vi "Receive Value Change Event.vi"(8 "error in (no error)":errorcluster, 10 "ValueChangeMsg":refnum<class "ValueChangeMsg.lvclass">, 11 "Login View In":refnum<class "Login View.lvclass">) -> (0 "error out":errorcluster, 3 "Login View Out":refnum<class "Login View.lvclass">)   [LabVIEW 2017, in "Login View.lvlib" / "Login View.lvclass"]
doc: "<License>\nCopyright © 2017 Composed Systems, LLC | All rights reserved\nwww.composed.io\n\nAuthor: Ethan Stern <ethan.stern@composed.io>\n\nThis software is provided \"AS IS\" WITHOUT WARRANTIES, either express or implied, AND IS FOR EDUCATIONAL PURPOSES ONLY.\n</License>"
uses:
  Login View.lvclass
  <vilib>/gpm_packages/@cs/mva-viewable/Source/ActorEvents/IEventAggregator Messages/ValueChangeMsg/ValueChangeMsg.lvclass
  <vilib>/gpm_packages/@cs/mva-viewable/Source/ActorEvents/IEventAggregator Messages/ValueChangeMsg/ValueChangeMsg.lvclass/ValueChangeMsg.ctl
  Login View.lvclass/Login View.ctl
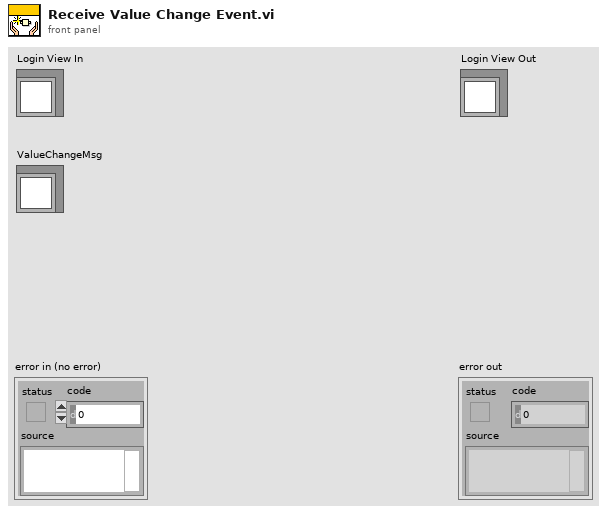
[diagram p1: front panel]
types:
  T1 = typedef "User Manager Application Types.lvlib/Credentials.ctl" = cluster{"Username":string, "Password":string}
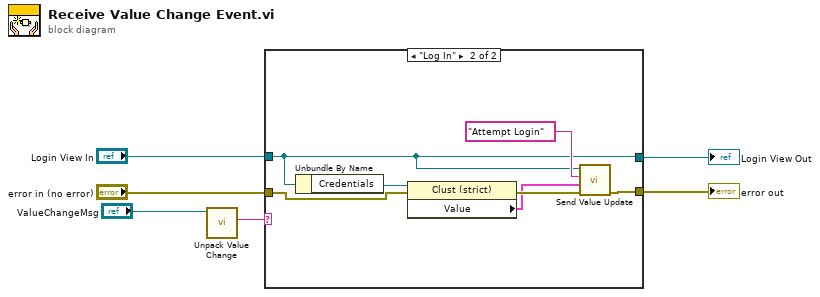
[diagram p0: block diagram]
diagram:
  n1 = call <vilib>:"Unpack Value Change.vi"("ValueChangeMsg"="ValueChangeMsg") -> ("Control Label"=w1:string)  [unwired: 6 in, 4 out]
  n2 = case shown="\"Log In\"" w1 {
    tunnel: [w7 w15] -> w6
    tunnel: [w8 w13] -> w5
    tunnel: "error in (no error)" -> [w7 w10]
    tunnel: "Login View In" -> [w8 w13]
    frame "False", Default {
    }
    frame "Log In" {
      n3 = Unbundle By Name(w13) -> ("Credentials"=w12:refnum<vi>)
      n4 = property class="Clust (strict)"(reference=w12, error in=w10) -> (error out=w11:errorcluster, "Value"=w9:T1)  [unwired: 1 out]
      n5 = call-dynamic "Send Value Update.vi"("error in (no error)"=w11, "Value"=w9, "Datum Name"="Attempt Login", "IViewable in"=w13) -> ("error out"=w15:errorcluster)  [unwired: 7 in]
    }
  }
  "error out" <- w6
  "Login View Out" <- w5
